vi "baogao4.vi"() -> ()   [LabVIEW 2017]
panel:
  out "dt":i32
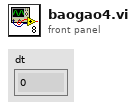
[diagram p1: front panel]
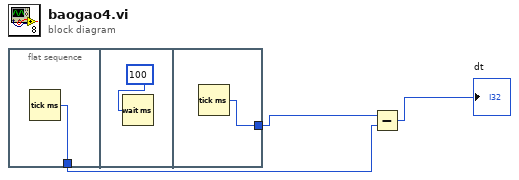
[diagram p0: block diagram]
diagram:
  n1 = flat-sequence {
    tunnel: [w4] -> w1
    tunnel: [w6] -> w2
    frame #0 {
      n2 = Tick Count (ms)() -> (millisecond timer value=w4:u32)
    }
    frame #1 {
      n3 = Wait (ms)(milliseconds to wait=100) -> ()  [unwired: 1 out]
    }
    frame #2 {
      n4 = Tick Count (ms)() -> (millisecond timer value=w6:u32)
    }
  }
  n5 = Subtract(x=w2, y=w1) -> (x-y=→"dt":u32)
